vi "final.vi"() -> ()   [LabVIEW 2022 SP3]
uses:
  <vilib>/DAQmx/read.llb/DAQmx Read (Analog 1D DBL NChan 1Samp).vi
  <vilib>/DAQmx/write.llb/DAQmx Write (Digital Bool 1Line 1Point).vi
  <vilib>/DAQmx/create/channels.llb/DAQmx Create Channel (AI-Voltage-Basic).vi
  <vilib>/DAQmx/create/channels.llb/DAQmx Create Channel (DO-Digital Output).vi
  <vilib>/DAQmx/miscellaneous.llb/DAQmx Fill In Error Info.vi
panel:
  out "voltage pulse from the Rpi":dbl
  in  "stop 2":bool
  in  "lines 5":tag
  in  "lines 4":tag
  in  "lines 3":tag
  in  "lines 2":tag
  out "voltage (weight)":dbl
  out "weight":dbl
  out "number":dbl
  out "Counter":dbl
  out "?":bool
  in  "Voltage":dbl
  out "humidity":dbl
  in  "lines":tag
  in  "physical channels":tag
  in  "stop":bool
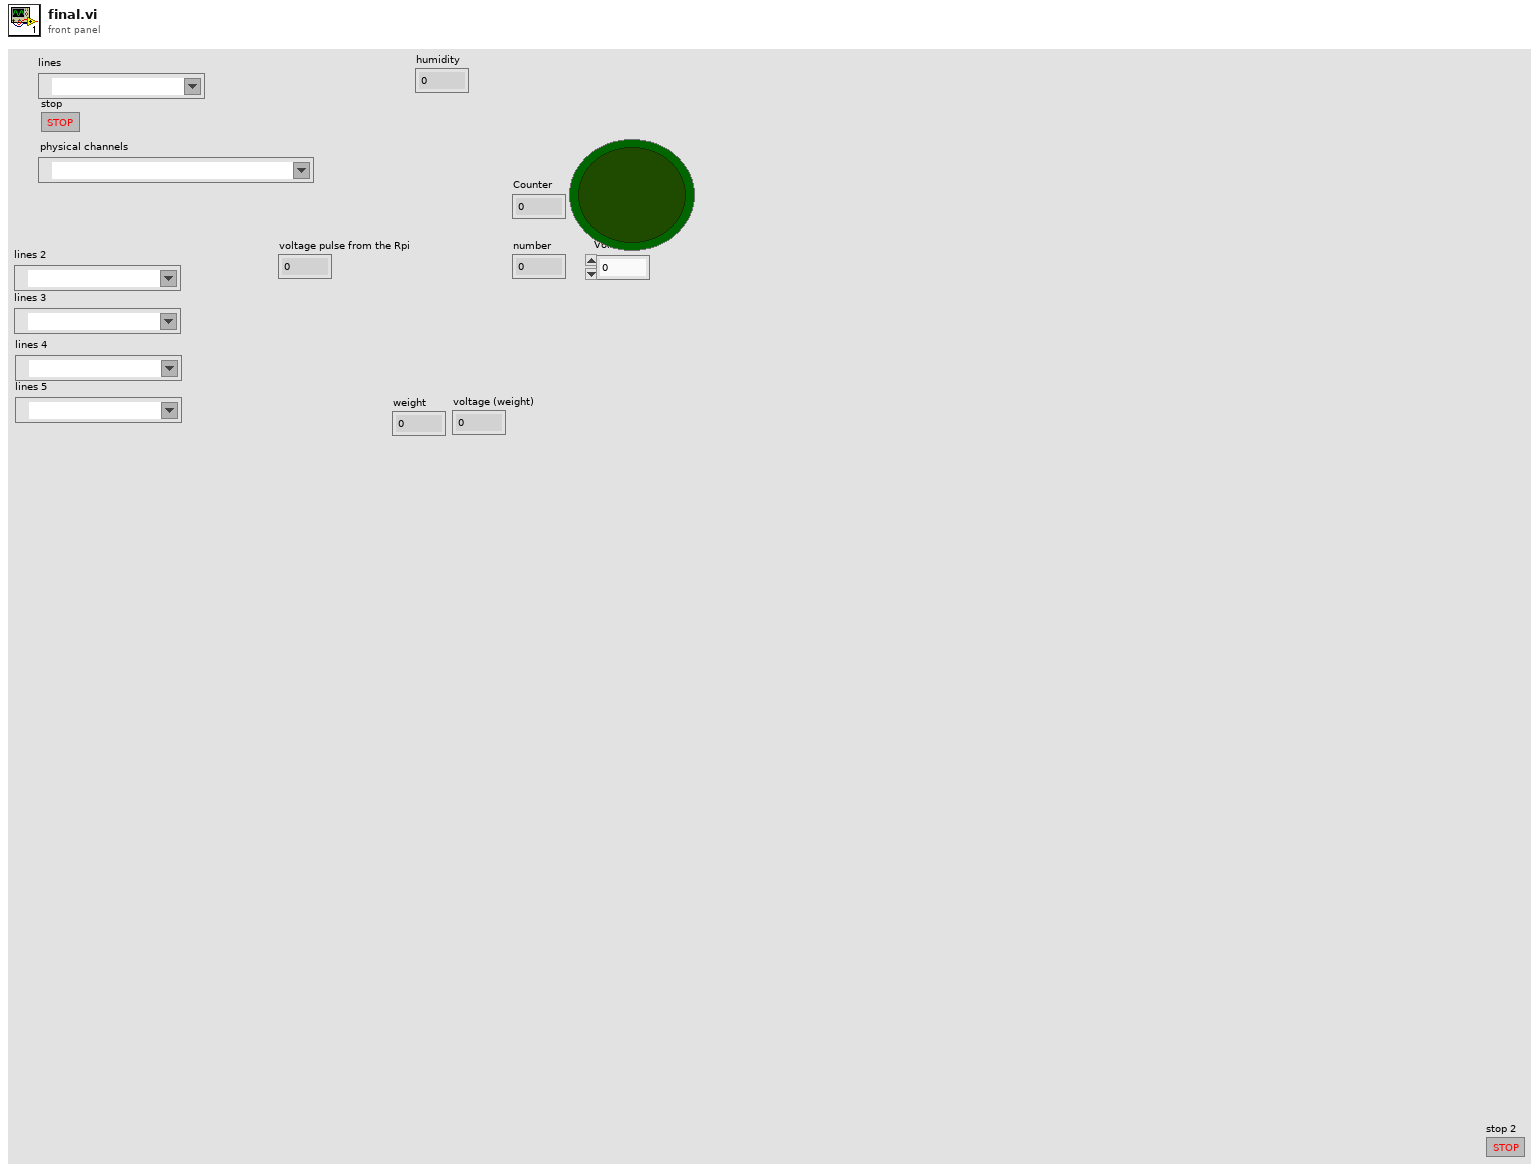
[diagram p1: front panel]
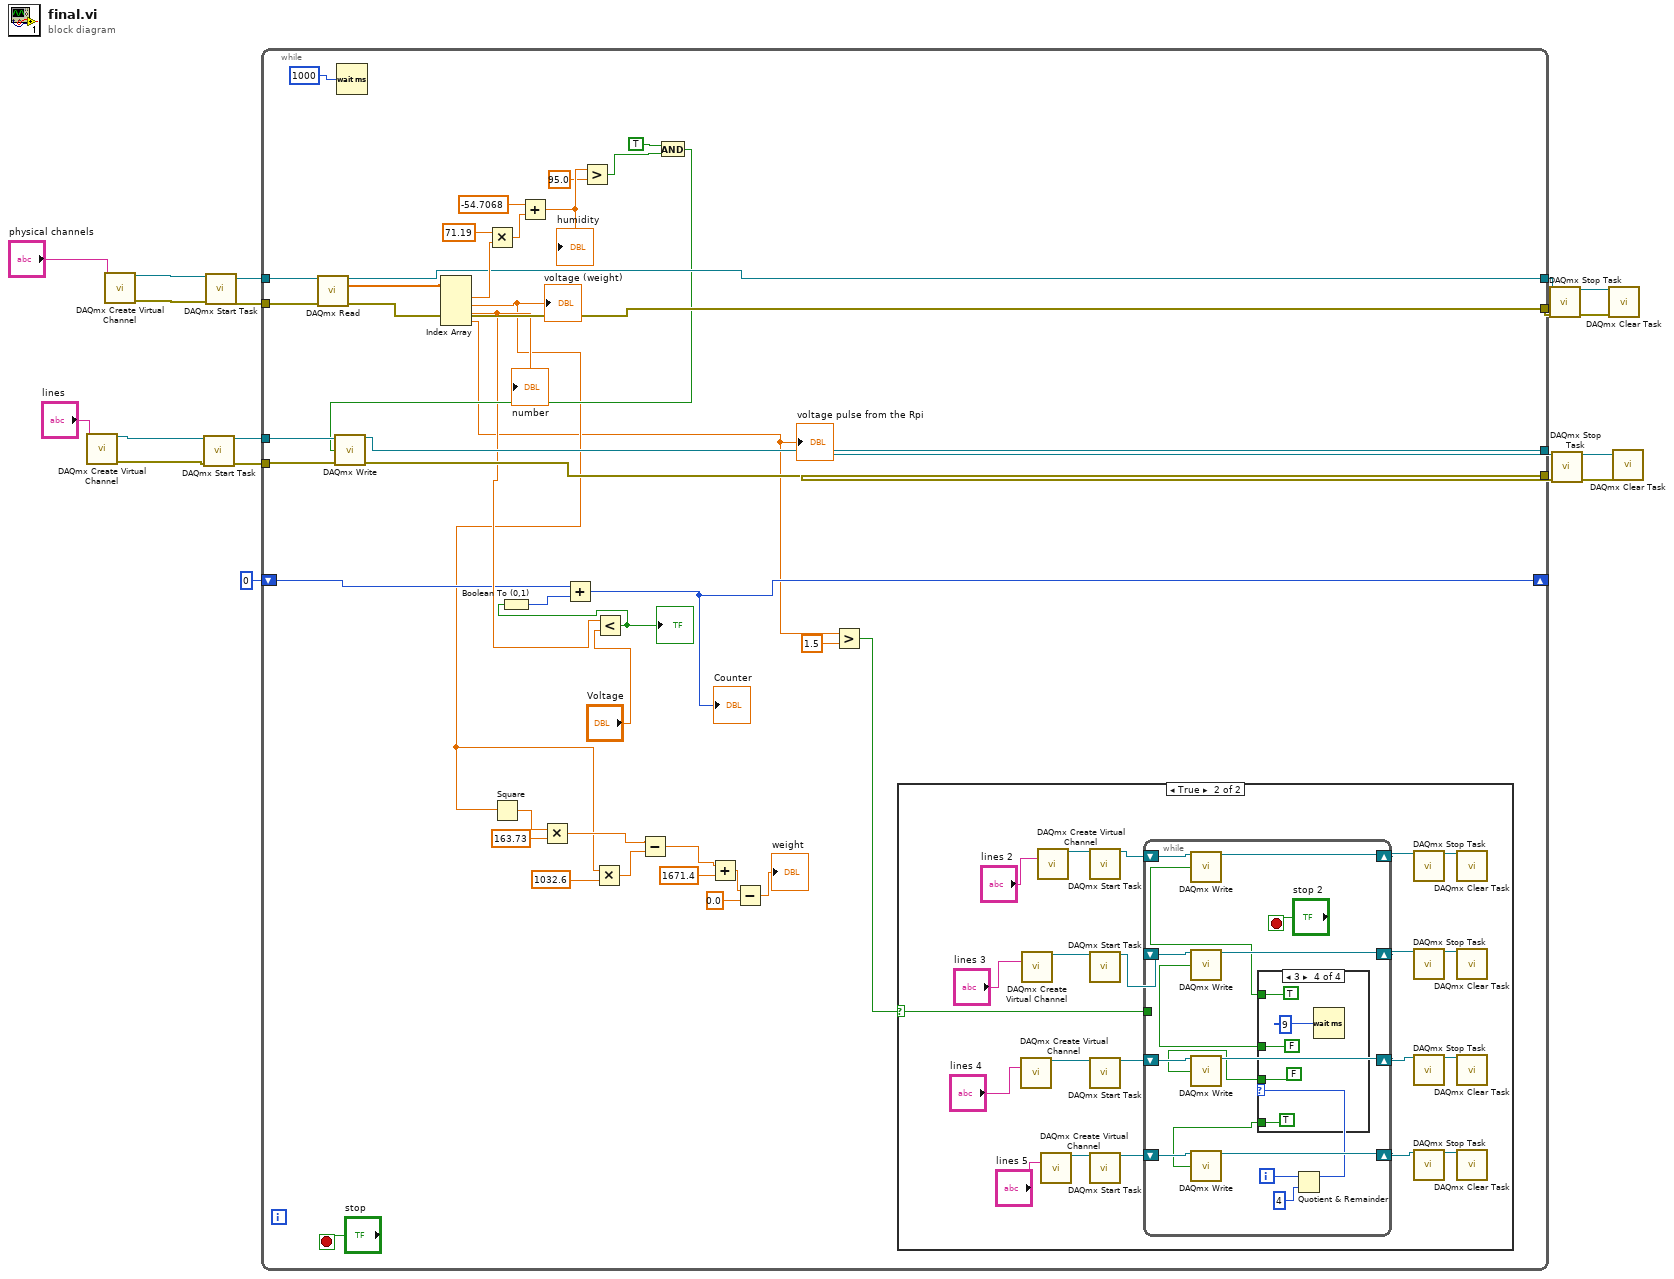
[diagram p0: block diagram]
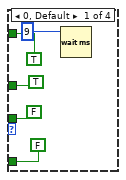
[diagram p3: hidden frame]
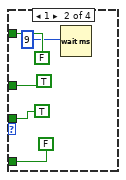
[diagram p4: hidden frame]
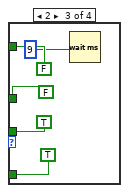
[diagram p5: hidden frame]
diagram:
  n1 = call-poly <vilib>:"DAQmx Create Virtual Channel.vi"("lines"="lines") -> ("task out"=w11:refnum<k21>, "error out"=w9:errorcluster)  [unwired: 13 in]
  n2 = call-poly <vilib>:"DAQmx Create Virtual Channel.vi"("physical channels"="physical channels") -> ("task out"=w19:refnum<k21>, "error out"=w18:errorcluster)  [unwired: 13 in]
  n3 = call <vilib>:"DAQmx Start Task.vi"("task/channels in"=w11, "error in"=w9) -> ("task out"=w10:refnum<k21>, "error out"=w8:errorcluster)  [unwired: 12 in]
  n4 = call <vilib>:"DAQmx Start Task.vi"("task/channels in"=w19, "error in"=w18) -> ("task out"=w17:refnum<k21>, "error out"=w16:errorcluster)  [unwired: 12 in]
  n5 = while {
    tunnel: w17 -> [w59]
    tunnel: w16 -> [w58]
    tunnel: [w42] -> w15
    tunnel: w10 -> [w48]
    tunnel: w8 -> [w44]
    tunnel: [w47] -> w7
    tunnel: [w46] -> w6
    tunnel: [w43] -> w3
    shift-right: [w35] -> _
    shift-left: i16 0 -> [w34]
    stop <- "stop" stop-if-true
    n6 = call-poly <vilib>:"DAQmx Read.vi"("task/channels in"=w59, "error in"=w58) -> ("task out"=w42:refnum<k21>, "data"=w55:dbl[], "error out"=w43:errorcluster)  [unwired: 11 in]
    n7 = Wait (ms)(milliseconds to wait=u32 1000) -> ()  [unwired: 1 out]
    n8 = Index Array(array=w55) -> (element #1=w53:dbl, element #2=w26:dbl, element #3=w36:dbl, element #4=w22:dbl)  [unwired: 4 in]
    "number" <- w36
    "voltage (weight)" <- w26
    "voltage pulse from the Rpi" <- w22
    n9 = Multiply(x=71.19, y=w53) -> (x*y=w54:dbl)
    n10 = Square(x=w26) -> (x^2=w33:dbl)
    n11 = Add(x=-54.7068, y=w54) -> (x+y=w52:dbl)
    "humidity" <- w52
    n12 = Multiply(x=w33, y=163.73) -> (x*y=w30:dbl)
    n13 = Greater?(x=w52, y=95.0) -> (0:w50:bool)
    n14 = Multiply(x=w26, y=1032.6) -> (x*y=w29:dbl)
    n15 = Less?(x=w36, y="Voltage") -> (x < y?=w37:bool)
    "?" <- w37
    n16 = Boolean To (0,1)(Boolean=w37) -> (0, 1=w38:i16)
    n17 = Add(x=w34, y=w38) -> (x+y=w35:i16)
    "Counter" <- w35
    n18 = Subtract(x=w30, y=w29) -> (x-y=w27:dbl)
    n19 = And(x=TRUE, y=w50) -> (x .and. y?=w41:bool)
    n20 = call-poly <vilib>:"DAQmx Write.vi"("task/channels in"=w48, "data"=w41, "error in"=w44) -> ("task out"=w47:refnum<k21>, "error out"=w46:errorcluster)  [unwired: 10 in, 1 out]
    n21 = Add(x=w27, y=1671.4) -> (x+y=w24:dbl)
    n22 = Subtract(x=w24, y=0.0) -> (x-y=→"weight":dbl)
    n23 = Greater?(x=w22, y=1.5) -> (0:w20:bool)
    n24 = case shown="True" w20 {
      selector: w20 -> [_ w60]
      frame False {
      }
      frame True {
        n25 = call-poly <vilib>:"DAQmx Create Virtual Channel.vi"("lines"="lines 4") -> ("task out"=w70:refnum<k21>)  [unwired: 13 in, 1 out]
        n26 = call-poly <vilib>:"DAQmx Create Virtual Channel.vi"("lines"="lines 3") -> ("task out"=w75:refnum<k21>)  [unwired: 13 in, 1 out]
        n27 = call-poly <vilib>:"DAQmx Create Virtual Channel.vi"("lines"="lines 2") -> ("task out"=w80:refnum<k21>)  [unwired: 13 in, 1 out]
        n28 = call-poly <vilib>:"DAQmx Create Virtual Channel.vi"("lines"="lines 5") -> ("task out"=w65:refnum<k21>)  [unwired: 13 in, 1 out]
        n29 = call <vilib>:"DAQmx Start Task.vi"("task/channels in"=w80) -> ("task out"=w79:refnum<k21>)  [unwired: 13 in, 1 out]
        n30 = call <vilib>:"DAQmx Start Task.vi"("task/channels in"=w75) -> ("task out"=w74:refnum<k21>)  [unwired: 13 in, 1 out]
        n31 = call <vilib>:"DAQmx Start Task.vi"("task/channels in"=w70) -> ("task out"=w69:refnum<k21>)  [unwired: 13 in, 1 out]
        n32 = call <vilib>:"DAQmx Start Task.vi"("task/channels in"=w65) -> ("task out"=w64:refnum<k21>)  [unwired: 13 in, 1 out]
        n33 = while {
          shift-right: [w95] -> w77
          shift-left: w79 -> [w96]
          shift-right: [w93] -> w72
          shift-left: w74 -> [w94]
          shift-right: [w91] -> w67
          shift-left: w69 -> [w92]
          shift-right: [w89] -> w62
          shift-left: w64 -> [w90]
          tunnel: w60 -> [_]
          i -> [w87]
          stop <- "stop 2" stop-if-true
          n34 = Quotient & Remainder(x=w87, y=4) -> (x-y*floor(x/y)=w81:i32)  [unwired: 1 out]
          n35 = case shown="3" w81 {
            tunnel: [TRUE FALSE FALSE TRUE] -> w85
            tunnel: [TRUE TRUE FALSE FALSE] -> w84
            tunnel: [FALSE TRUE TRUE FALSE] -> w83
            tunnel: [FALSE FALSE TRUE TRUE] -> w82
            frame 0, Default {
              n36 = Wait (ms)(milliseconds to wait=9) -> ()  [unwired: 1 out]
            }
            frame 1 {
              n37 = Wait (ms)(milliseconds to wait=9) -> ()  [unwired: 1 out]
            }
            frame 2 {
              n38 = Wait (ms)(milliseconds to wait=9) -> ()  [unwired: 1 out]
            }
            frame 3 {
              n39 = Wait (ms)(milliseconds to wait=9) -> ()  [unwired: 1 out]
            }
          }
          n40 = call-poly <vilib>:"DAQmx Write.vi"("task/channels in"=w96, "data"=w85) -> ("task out"=w95:refnum<k21>)  [unwired: 11 in, 2 out]
          n41 = call-poly <vilib>:"DAQmx Write.vi"("task/channels in"=w94, "data"=w84) -> ("task out"=w93:refnum<k21>)  [unwired: 11 in, 2 out]
          n42 = call-poly <vilib>:"DAQmx Write.vi"("task/channels in"=w92, "data"=w83) -> ("task out"=w91:refnum<k21>)  [unwired: 11 in, 2 out]
          n43 = call-poly <vilib>:"DAQmx Write.vi"("task/channels in"=w90, "data"=w82) -> ("task out"=w89:refnum<k21>)  [unwired: 11 in, 2 out]
        }
        n44 = call <vilib>:"DAQmx Stop Task.vi"("task/channels in"=w77) -> ("task out"=w78:refnum<k21>)  [unwired: 13 in, 1 out]
        n45 = call <vilib>:"DAQmx Stop Task.vi"("task/channels in"=w72) -> ("task out"=w73:refnum<k21>)  [unwired: 13 in, 1 out]
        n46 = call <vilib>:"DAQmx Stop Task.vi"("task/channels in"=w67) -> ("task out"=w68:refnum<k21>)  [unwired: 13 in, 1 out]
        n47 = call <vilib>:"DAQmx Stop Task.vi"("task/channels in"=w62) -> ("task out"=w63:refnum<k21>)  [unwired: 13 in, 1 out]
        n48 = call <vilib>:"DAQmx Clear Task.vi"("task in"=w78) -> ()  [unwired: 14 in, 1 out]
        n49 = call <vilib>:"DAQmx Clear Task.vi"("task in"=w73) -> ()  [unwired: 14 in, 1 out]
        n50 = call <vilib>:"DAQmx Clear Task.vi"("task in"=w68) -> ()  [unwired: 14 in, 1 out]
        n51 = call <vilib>:"DAQmx Clear Task.vi"("task in"=w63) -> ()  [unwired: 14 in, 1 out]
      }
    }
  }
  n52 = call <vilib>:"DAQmx Stop Task.vi"("task/channels in"=w15, "error in"=w3) -> ("task out"=w13:refnum<k21>, "error out"=w14:errorcluster)  [unwired: 12 in]
  n53 = call <vilib>:"DAQmx Stop Task.vi"("task/channels in"=w7, "error in"=w6) -> ("task out"=w5:refnum<k21>, "error out"=w4:errorcluster)  [unwired: 12 in]
  n54 = call <vilib>:"DAQmx Clear Task.vi"("task in"=w13, "error in"=w14) -> ()  [unwired: 13 in, 1 out]
  n55 = call <vilib>:"DAQmx Clear Task.vi"("task in"=w5, "error in"=w4) -> ()  [unwired: 13 in, 1 out]
